vi "flat_Secunce.vi"() -> ()   [LabVIEW 2020]
panel:
  in  "stop":bool
  out "Boolean 2":bool
  in  "Boolean":bool
  out "Array":i32[](array[numeric])
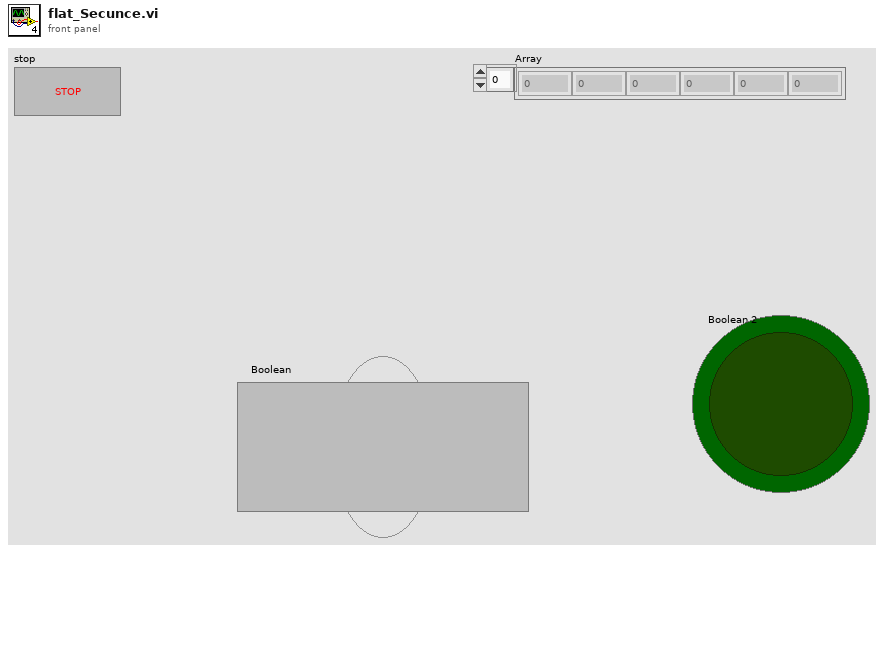
[diagram p1: front panel]
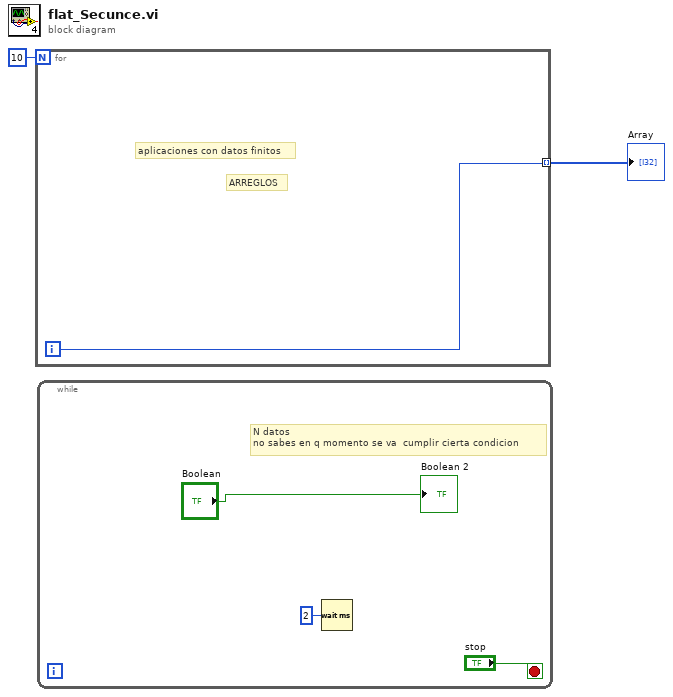
[diagram p0: block diagram]
diagram:
  n1 = for {
    N: 10 -> [_]
    tunnel: [w3] -> w2 mode=indexing
    i -> [w3]
    # "ARREGLOS"
    # "aplicaciones con datos finitos"
  }
  "Array" <- w2
  n2 = while {
    stop <- "stop" stop-if-true
    # "N datos\nno sabes en q momento se va  cumplir cierta condicion"
    n3 = Wait (ms)(milliseconds to wait=u32 2) -> ()  [unwired: 1 out]
    "Boolean 2" <- "Boolean"
  }
